vi "Global - Name of loaded Module.vi"() -> ()   [LabVIEW 2019, in "Subpanel Tools.lvlib"]
uses:
  Subpanel Tools.lvlib
panel:
  in  "Name of loaded Modle":string
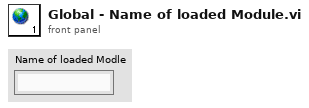
[diagram p1: front panel]
diagram:
